vi "Load Configuration.vi"(7 "Cursor Already Busy?":bool, 8 "error in (no error)":errorcluster, 10 "Config File to Load":path, 11 "Cfg Grandmaster in":refnum<class "Cfg Grandmaster.lvclass">) -> (0 "error out":errorcluster, 3 "Cfg Grandmaster out":refnum<class "Cfg Grandmaster.lvclass">)   [LabVIEW 2012, in "Configuration Grandmaster.lvlib" / "Cfg Grandmaster.lvclass"]
uses:
  Cfg Grandmaster.lvclass
  Cfg Grandmaster.lvclass/Cfg Grandmaster.ctl
  Class Chassis BOM/Chassis BOM.lvclass/Chassis BOM.ctl
  Class Chassis BOM/Read Chassis Alias.vi
  Class Chassis BOM/Chassis BOM.lvclass
  Class FP Ctrls/FP Controls.lvclass
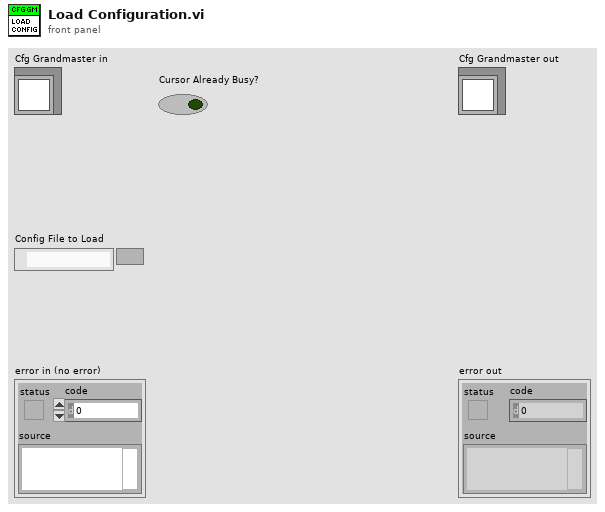
[diagram p1: front panel]
types:
  T1 = typedef "ge_Cfg wChassis.ctl" = cluster{"Chassis BOM":refnum<class "Chassis BOM.lvclass">, "Chassis Cfg":refnum<class "ChassisCfg.lvclass">, "Chassis Tasks":refnum<class "Chassis Tasks.lvclass">, "HW Error":bool, "Unsvd Chgs?":bool}
  T2 = typedef "Selected Group.ctl" = cluster{"ChanGroup":i32, "Rate Class":T3}
  T3 = typedef "TE_Designator.ctl" = enum16{"High Speed", "Low Speed"}
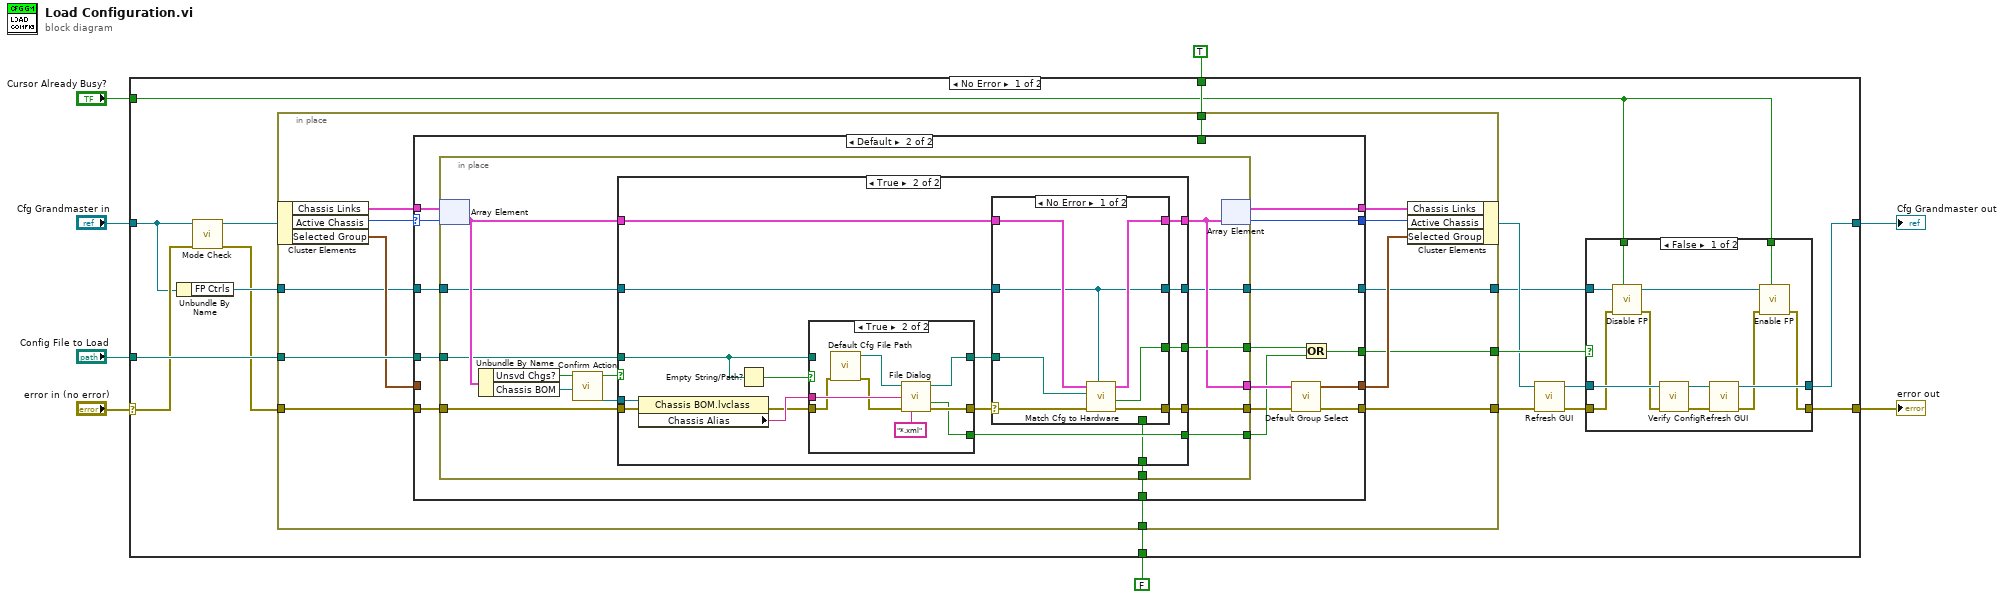
[diagram p0: block diagram]
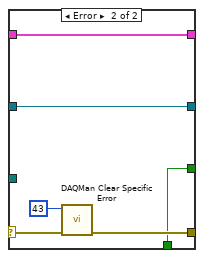
[diagram p6: hidden frame]
diagram:
  n1 = case shown="No Error" "error in (no error)" {
    selector: "error in (no error)" -> [w22 w134]
    tunnel: [w11 w134] -> w7
    tunnel: [w19 w133] -> w5
    tunnel: "Cfg Grandmaster in" -> [w18 w133]
    tunnel: "Config File to Load" -> [w25 _]
    tunnel: TRUE -> [w24 _]
    tunnel: FALSE ("HW Error?") -> [w21 _]
    tunnel: "Cursor Already Busy?" -> [w9 _]
    frame No Error {
      n2 = Unbundle By Name(w18) -> ("FP Ctrls"=w13:refnum<class "FP Controls.lvclass">)
      n3 = call "Mode Check.vi"("error in (no error)"=w22, "Cfg Grandmaster in"=w18) -> ("error out"=w12:errorcluster, "Cfg Grandmaster out"=w23:refnum<class "Cfg Grandmaster.lvclass">)  [unwired: 8 in]
      n4 = in-place {
        in-place-border: w12 -> [w53]
        in-place-border: w25 -> [w52]
        in-place-border: [w51] -> w15
        in-place-border: w24 -> [w44]
        in-place-border: [w43] -> w20
        in-place-border: w21 -> [w42]
        in-place-border: w13 -> [w41]
        in-place-border: [w40] -> w10
        n5 = in-place-cluster #1(w23) -> ("Chassis Links"=w50:T1[], "Active Chassis"=w46:i32, "Selected Group"=w45:T2)
        n6 = case shown="Default" w46 {
          selector: w46 -> [w56 w67]
          tunnel: [w58 w69] -> w51
          tunnel: [w59 w66] -> w49
          tunnel: w50 -> [w59 w68]
          tunnel: [w57 w74] -> w48
          tunnel: [w55 w71] -> w43
          tunnel: w53 -> [w58 w62]
          tunnel: w52 -> [_ w65]
          tunnel: w45 -> [w57 _]
          tunnel: [w56 w64] -> w47
          tunnel: w44 -> [w55 _]
          tunnel: w42 -> [_ w63]
          tunnel: w41 -> [w54 w61]
          tunnel: [w54 w60] -> w40
          frame -1 {
          }
          frame Default {
            n7 = in-place {
              in-place-border: [w85] -> w75
              in-place-border: [w88] -> w73
              in-place-border: [w87] -> w72
              in-place-border: w65 -> [w81]
              in-place-border: w62 -> [w82]
              in-place-border: [w86] -> w70
              in-place-border: w63 -> [w78]
              in-place-border: w61 -> [w77]
              in-place-border: [w76] -> w60
              n8 = in-place-array #2(w68, w67) -> (w84:T1)
              n9 = Unbundle By Name(w84) -> ("Unsvd Chgs?"=w80:bool, "Chassis BOM"=w83:refnum<class "Chassis BOM.lvclass">)
              n10 = call "Confirm Action.vi"("Confirm?"=w80) -> ("T button?"=w79:bool)  [unwired: 10 in]
              n11 = case shown="True" w79 {
                tunnel: [w90 w106] -> w88
                tunnel: [w90 w105] -> w87
                tunnel: [w91 w104] -> w86
                tunnel: [w92 w103] -> w85
                tunnel: w84 -> [w92 w101]
                tunnel: w83 -> [_ w100]
                tunnel: w82 -> [w91 w98]
                tunnel: w81 -> [_ w96]
                tunnel: w78 -> [w90 w97]
                tunnel: w77 -> [w89 w94]
                tunnel: [w89 w93] -> w76
                frame False {
                }
                frame True {
                  n12 = property class="Chassis BOM.lvclass"(reference=w100, error in=w98) -> (error out=w99:errorcluster, "Chassis Alias"=w102:string)  [unwired: 1 out]
                  n13 = Empty String/Path?(string/path=w96) -> (empty?=w95:bool)
                  n14 = case shown="True" w95 {
                    selector: w95 -> [w109 _]
                    tunnel: [w110 w119] -> w108
                    tunnel: [w111 w118] -> w107
                    tunnel: w96 -> [w110 _]
                    tunnel: w99 -> [w111 w113]
                    tunnel: [w109 w117] -> w105
                    tunnel: w102 -> [_ w115]
                    frame False {
                    }
                    frame True {
                      n15 = call "Default Cfg File Path.vi"("error in (no error)"=w113) -> ("error out"=w112:errorcluster, "Default Path"=w114:path)  [unwired: 9 in]
                      n16 = call "File Dialog"("start path"=w114, "default name"=w115, "error in"=w112, "pattern (all files)"="*.xml") -> ("selected path"=w119:path, "cancelled"=w117:bool, "error out"=w118:errorcluster)  [unwired: 8 in, 1 out]
                    }
                  }
                  n17 = case shown="No Error" w107 {
                    selector: w107 -> [w126 w131]
                    tunnel: [w124 w129] -> w104
                    tunnel: w108 -> [w121 _]
                    tunnel: w101 -> [w122 w130]
                    tunnel: [w123 w130] -> w103
                    tunnel: [w125 w128] -> w106
                    tunnel: w97 -> [_ w128]
                    tunnel: w94 -> [w120 w127]
                    tunnel: [w120 w127] -> w93
                    frame No Error {
                      n18 = call "Match Cfg to Hardware.vi"("FP Ctrls"=w120, "error in"=w126, "selected path"=w121, "Cfg wChassis"=w122) -> ("error out"=w124:errorcluster, "HW Error?"=w125:bool, "Cfg wChassis"=w123:T1)  [unwired: 5 in]
                    }
                    frame Error {
                      n19 = call "DAQMan Clear Specific Error.vi"("error in"=w131, "code"=43 ("y")) -> ("error out"=w129:errorcluster)  [unwired: 9 in]
                    }
                  }
                }
              }
              n20 = in-place-array #2(w85) -> (w66:T1[], w64:i32)
            }
            n21 = call "Default Group Select.vi"("error in"=w70, "Cfg with Chassis"=w75) -> ("error out"=w69:errorcluster, "Selected Grp"=w74:T2)  [unwired: 8 in]
            n22 = Or(x=w73, y=w72) -> (x .or. y?=w71:bool)
          }
        }
        n23 = in-place-cluster #1("Chassis Links"=w49, "Active Chassis"=w47, "Selected Group"=w48) -> (w14:refnum<class "Cfg Grandmaster.lvclass">)
      }
      n24 = call "Refresh GUI.vi"("error in (no error)"=w15, "Cfg Grandmaster in"=w14) -> ("error out"=w16:errorcluster, "Cfg Grandmaster out"=w17:refnum<class "Cfg Grandmaster.lvclass">)  [unwired: 8 in]
      n25 = case shown="False" w20 {
        tunnel: [w28 w39] -> w11
        tunnel: w16 -> [w31 w39]
        tunnel: w17 -> [w34 w38]
        tunnel: [w35 w38] -> w19
        tunnel: w10 -> [w33 _]
        tunnel: w9 -> [w27 _]
        tunnel: w9 -> [w26 _]
        frame False {
          n26 = call "Disable FP.vi"("Ignore?"=w27, "error in (no error)"=w31, "FP Controls in"=w33) -> ("error out"=w30:errorcluster, "FP Controls out"=w32:refnum<class "FP Controls.lvclass">)  [unwired: 7 in]
          n27 = call "Verify Config.vi"("error in (no error)"=w30, "Cfg Grandmaster in"=w34) -> ("error out"=w37:errorcluster, "Cfg Grandmaster out"=w36:refnum<class "Cfg Grandmaster.lvclass">)  [unwired: 8 in]
          n28 = call "Refresh GUI.vi"("error in (no error)"=w37, "Cfg Grandmaster in"=w36) -> ("error out"=w29:errorcluster, "Cfg Grandmaster out"=w35:refnum<class "Cfg Grandmaster.lvclass">)  [unwired: 8 in]
          n29 = call "Enable FP.vi"("Ignore?"=w26, "error in (no error)"=w29, "FP Controls in"=w32) -> ("error out"=w28:errorcluster)  [unwired: 7 in, 1 out]
        }
        frame True {
        }
      }
    }
    frame Error {
    }
  }
  "error out" <- w7
  "Cfg Grandmaster out" <- w5
